vi "LSX Put Slide.vi"(8 "error in (no error)":errorcluster, 9 "slot":i32, 10 "maga":i32, 11 "lLSID":i32) -> (0 "error out":errorcluster, 3 "function return":i32)   [LabVIEW 2018, in "Tango.lvlib"]
doc: "TANGOAPI int TANGOCALL LSX_PutSlide (int lLSID, int maga, int slot);"
uses:
  <userlib>/Tango/Tango.lvlib
  <userlib>/Tango/Tango_DLL.dll
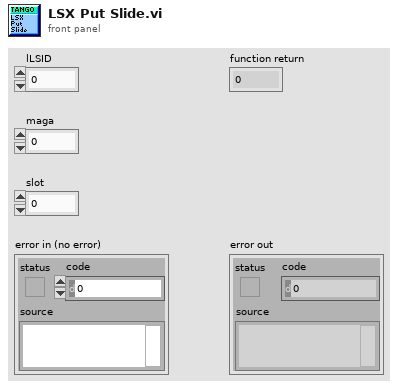
[diagram p1: front panel]
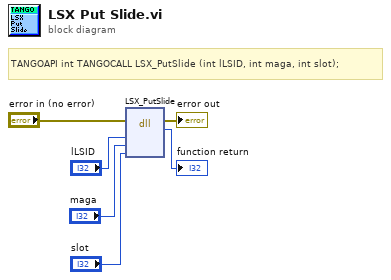
[diagram p0: block diagram]
diagram:
  # "TANGOAPI int TANGOCALL LSX_PutSlide (int lLSID, int maga, int slot);"
  n1 = dll-call lib="C:/Program Files (x86)/National Instruments/LabVIEW 2018/user.lib/Tango/Tango_DLL.*" fn="LSX_PutSlide"(error in="error in (no error)", "lLSID"="lLSID", "maga"="maga", "slot"="slot") -> (error out=→"error out":errorcluster, →"function return":i32)  [unwired: 5 in, 1 out]
